vi "Select Parents.vi"(6 "Target Chromosome":refnum<class "IChromosome.lvclass">, 8 "error in":errorcluster, 11 "IPopulation in":refnum<class "IPopulation.lvclass">) -> (0 "error out":errorcluster, 3 "IPopulation out":refnum<class "IPopulation.lvclass">)   [LabVIEW 2016, in "IPopulation.lvclass"]
uses:
  IPopulation.lvclass
  IChromosome/IChromosome.lvclass
  IPopulation.lvclass/IPopulation.ctl
  IChromosome/IChromosome.lvclass/IChromosome.ctl
  <userlib>/_OpenG.lib/numeric/numeric.llb/Random Number Within Range - I32__ogtk.vi
  IGene/IGene.lvclass
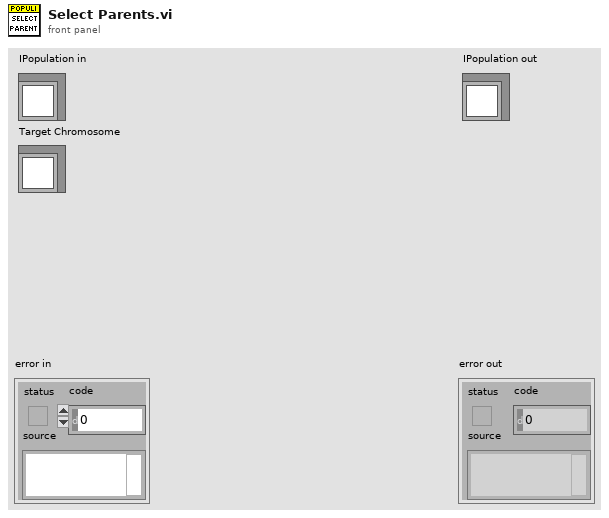
[diagram p1: front panel]
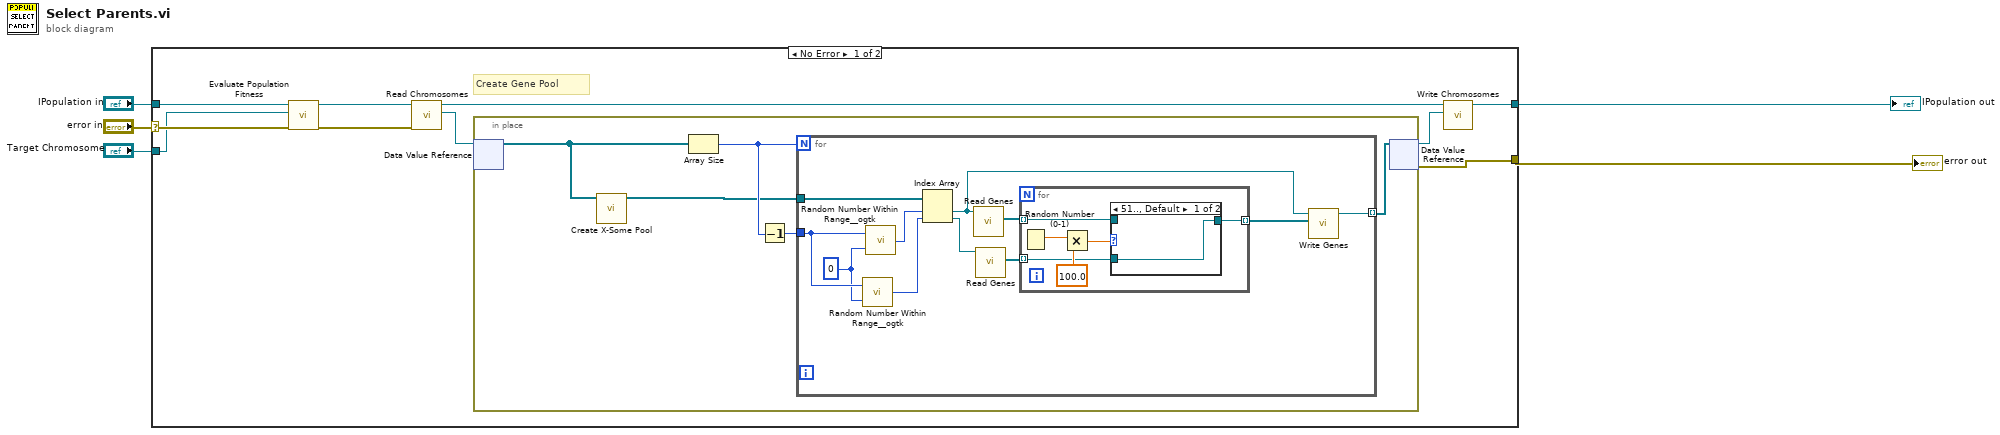
[diagram p0: block diagram]
diagram:
  n1 = case shown="No Error" "error in" {
    selector: "error in" -> [w14 w41]
    tunnel: [w9 w41] -> w4
    tunnel: [w6 w40] -> w2
    tunnel: "IPopulation in" -> [w15 w40]
    tunnel: "Target Chromosome" -> [w13 _]
    frame No Error {
      # "Create Gene Pool"
      n2 = call "Evaluate Population Fitness.vi"("error in"=w14, "Target Chromosome"=w13, "IPopulation in"=w15) -> ("error out"=w11:errorcluster, "IPopulation out"=w12:refnum<class "IPopulation.lvclass">)  [unwired: 7 in]
      n3 = call "Read Chromosomes.vi"("error in (no error)"=w11, "IPopulation in"=w12) -> ("Chromosomes"=w10:refnum<data-value>, "IPopulation out"=w8:refnum<class "IPopulation.lvclass">)  [unwired: 7 in, 1 out]
      n4 = in-place {
        n5 = in-place-dvr #1(w10) -> (w17:refnum<class "IChromosome.lvclass">[])  [unwired: 1 out]
        n6 = call "Create X-Some Pool.vi"("Chromosomes In"=w17) -> ("X-Some Pool Out"=w16:refnum<class "IChromosome.lvclass">[])  [unwired: 10 in]
        n7 = Array Size(array=w17) -> (size(s)=w18:i32)
        n8 = Decrement(x=w18) -> (x-1=w20:i32)
        n9 = for {
          N: w18 -> [_]
          tunnel: w20 -> [w31]
          tunnel: w16 -> [w30]
          tunnel: [w23] -> w19 mode=indexing
          w21 = 0 ("Low")
          n10 = call-poly <userlib>:"Random Number Within Range__ogtk.vi"("High"=w31, "Low"=w21) -> ("Random Number"=w28:i32)  [unwired: 3 in]
          n11 = call-poly <userlib>:"Random Number Within Range__ogtk.vi"("High"=w31, "Low"=w21) -> ("Random Number"=w29:i32)  [unwired: 3 in]
          n12 = Index Array(array=w30, index #1=w29, index #2=w28) -> (element #1=w22:refnum<class "IChromosome.lvclass">, element #2=w27:refnum<class "IChromosome.lvclass">)
          n13 = call "Read Genes.vi"("IChromosome in"=w22) -> ("Genes"=w26:refnum<class "IGene.lvclass">[])  [unwired: 8 in, 2 out]
          n14 = call "Read Genes.vi"("IChromosome in"=w27) -> ("Genes"=w25:refnum<class "IGene.lvclass">[])  [unwired: 8 in, 2 out]
          n15 = for {
            tunnel: w26 -> [w34] mode=indexing
            tunnel: w25 -> [w33] mode=indexing
            tunnel: [w32] -> w24 mode=indexing
            n16 = Random Number (0-1)() -> (number: 0 to 1=w37:dbl)
            n17 = Multiply(x=w37, y=100.0) -> (x*y=w35:dbl)
            n18 = case shown="51.., Default" w35 {
              tunnel: w34 -> [_ w39]
              tunnel: w33 -> [w38 _]
              tunnel: [w38 w39] -> w32
              frame 51.., Default {
              }
              frame 0..50 {
              }
            }
          }
          n19 = call "Write Genes.vi"("Genes"=w24, "IChromosome in"=w22) -> ("IChromosome out"=w23:refnum<class "IChromosome.lvclass">)  [unwired: 8 in, 1 out]
        }
        n20 = in-place-dvr #1(w19) -> (w7:refnum<data-value>, w9:errorcluster)
      }
      n21 = call "Write Chromosomes.vi"("Chromosomes"=w7, "IPopulation in"=w8) -> ("IPopulation out"=w6:refnum<class "IPopulation.lvclass">)  [unwired: 8 in, 1 out]
    }
    frame Error {
    }
  }
  "error out" <- w4
  "IPopulation out" <- w2
